vi "Init.vi"(6 "Export Data Locations":string[](array[string]), 8 "error in (no error)":errorcluster, 9 "Harmonics":i8[](array[numeric]), 10 "Measurement Name":string, 11 "Standard":string) -> (0 "error out":errorcluster, 3 "Harmonics_Relative_Power out":refnum<class "Harmonics_Relative_Power.lvclass">)   [LabVIEW 2016, in "SeqAuto Evaluations.lvlib" / "Harmonics_Relative_Power.lvclass"]
uses:
  Harmonics_Relative_Power.lvclass
  C:/projects/STS/Common/Sequence Automation/Plugins/SeqAuto IEvaluation.lvlibp/SeqAuto IEvaluation.lvclass
  Harmonics_Relative_Power.lvclass/Harmonics_Relative_Power.ctl
  Write Export Data Locations.vi
  Write Harmonics.vi
  Plugins/SeqAuto IEvaluation.lvlibp/Write Measurement Name.vi
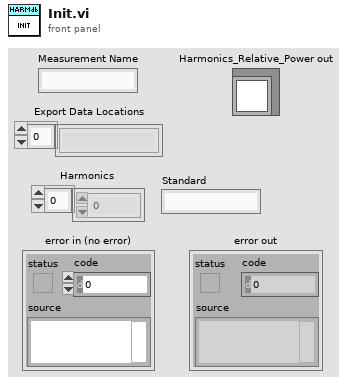
[diagram p1: front panel]
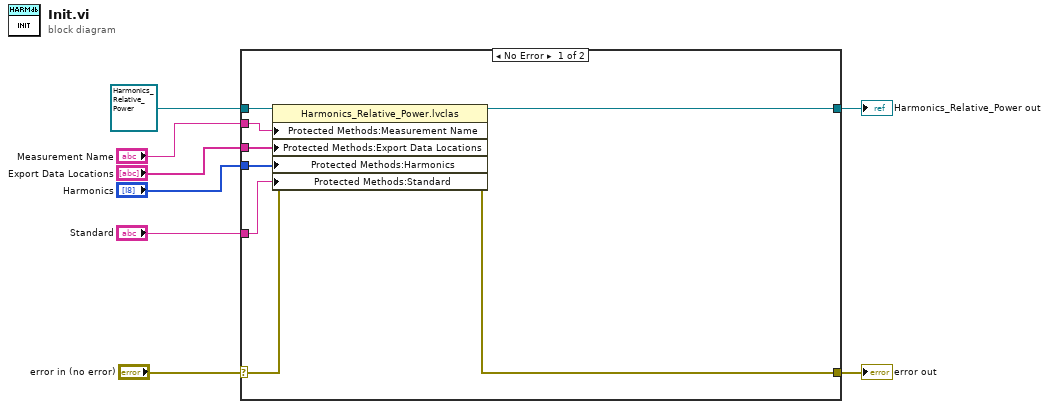
[diagram p0: block diagram]
diagram:
  n1 = case shown="No Error" "error in (no error)" {
    selector: "error in (no error)" -> [w16 w18]
    tunnel: [w15 w18] -> w7
    tunnel: [w9 w17] -> w5
    tunnel: refnum<class "Harmonics_Relative_Power.lvclass"> refnum ("Harmonics_Relative_Power in") -> [w14 w17]
    tunnel: "Measurement Name" -> [w13 _]
    tunnel: "Export Data Locations" -> [w12 _]
    tunnel: "Harmonics" -> [w11 _]
    tunnel: "Standard" -> [w10 _]
    frame No Error {
      n2 = property class="Harmonics_Relative_Power.lvclas"(reference=w14, error in=w16, "Protected Methods:Measurement Name"=w13, "Protected Methods:Export Data Locations"=w12, "Protected Methods:Harmonics"=w11, "Protected Methods:Standard"=w10) -> (reference out=w9:refnum<class "Harmonics_Relative_Power.lvclass">, error out=w15:errorcluster)
    }
    frame Error {
    }
  }
  "error out" <- w7
  "Harmonics_Relative_Power out" <- w5
